vi "Configure Hardware.vi"(8 "error in (no error)":errorcluster, 11 "Hardware Resources in":T1={"DO"={"task name"="AI", "task_ref"="", "lines"=""}}) -> (0 "error out":errorcluster, 3 "Hardware Resources out":T1={"DO"={"task name"="AI", "task_ref"="", "lines"=""}})   [LabVIEW 2014, in "PLS Digital Control.lvlib"]
doc: "Configure the hardware."
uses:
  PLS Digital Control.lvlib
  Hardware Configuration.ctl
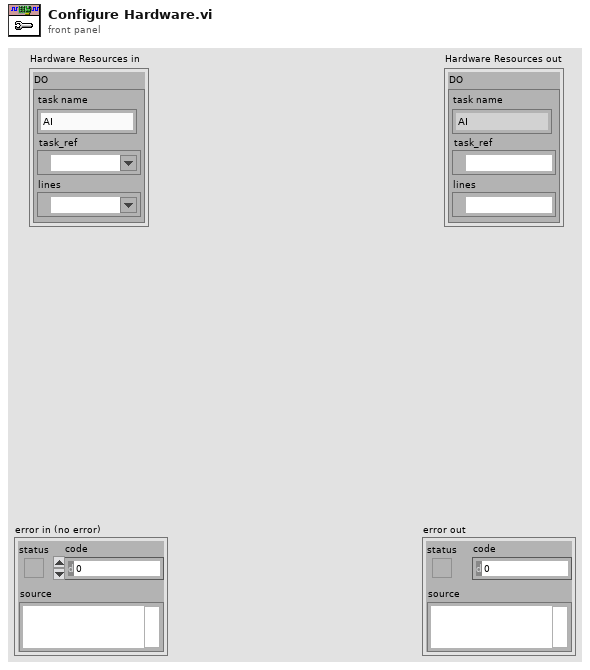
[diagram p1: front panel]
types:
  T1 = typedef "PLS Digital Control.lvlib/Hardware Configuration.ctl" = cluster{"DO":cluster{"task name":string, "task_ref":refnum<k21>, "lines":tag}}
  T2 = cluster{"task name":string, "task_ref":refnum<k21>, "lines":tag}
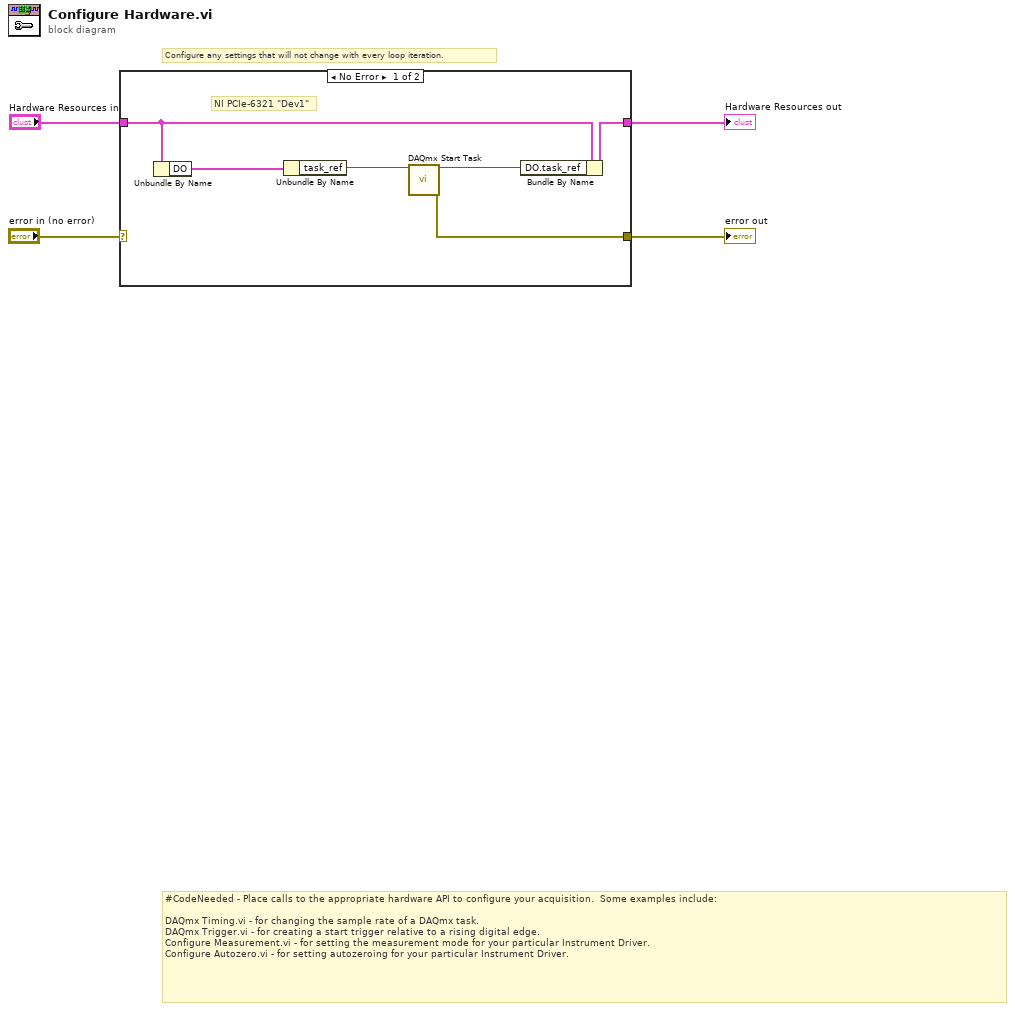
[diagram p0: block diagram]
diagram:
  # "Configure any settings that will not change with every loop iteration."
  # "#CodeNeeded - Place calls to the appropriate hardware API to configure your acquisition.  Some examples include:\n\nDAQmx Timing.vi - for changing the sample rate of a DAQmx task.\nDAQmx Trigger.vi - for creating a start trigger relative to a rising digital edge.\nConfigure Measurement.vi - for setting the measurement mode for your particular Instrument Driver.\nConfigure Autozero.vi - for setting autozeroing for your particular Instrument Driver."
  n1 = case shown="No Error" "error in (no error)" {
    selector: "error in (no error)" -> [_ w11]
    tunnel: [w5 w11] -> w3
    tunnel: "Hardware Resources in" -> [w8 w12]
    tunnel: [w10 w12] -> w1
    frame No Error {
      # "NI PCIe-6321 \"Dev1\""
      n2 = Unbundle By Name(w8) -> ("DO"=w6:T2)
      n3 = Unbundle By Name(w6) -> ("task_ref"=w7:refnum<k21>)
      n4 = call <vilib>:"DAQmx Start Task.vi"("task/channels in"=w7) -> ("task out"=w9:refnum<k21>, "error out"=w5:errorcluster)  [unwired: 13 in]
      n5 = Bundle By Name(cluster=w8, "DO.task_ref"=w9) -> (w10:T1)
    }
    frame Error {
    }
  }
  "Hardware Resources out" <- w1
  "error out" <- w3
